vi "SDG60ConfModulation.vi"(0 "VISA resource name":refnum<visa-resource-name>="USB0::0xF4EC::0x1101::SDG6XEBC5R0119::INSTR", 1 "Modulation Type (0: AM)":u16(ring) items=["AM", "FM", "PM", "PWM", "DSBAM", "ASK", "FSK", "PSK", "CARR"], 2 "Channel (1:Channel 1)":i32(ring)=1 items=["Channel 1"=1, "Channel 2"=2], 11 "error in (no error)":errorcluster) -> (4 "VISA resource name out":refnum<visa-resource-name>, 15 "error out":errorcluster)   [LabVIEW 2018]
doc: "Selects the waveform shape, frequency, amplitude, offset, and phase for standard waveforms (including Sine, Square, Ramp, Pulse, DC and Arb).\n\nNotes: \nTo configure other parameters for pulse waveforms please run the Configure Pulse VI. \nTo configure noise waveform please run the Configure Noise VI.\nTo configure other parameters for arbitrary waveforms please run the Create Arbitrary Waveform. \nTo configure PRBS waveform please run the Configure PRBS Waveform VI."
panel:
  in  "Phase (0 deg)":dbl format="%#_12g"
  in  "Depth (%)":dbl=1000.0 format="%#_16g"
  in  "Frequency (1 Hz)":dbl=1000.0 format="%#_16g"
  in  "Mod wave shape (0:Sine)":u16(ring) items=["Sine", "Square", "Triangle", "Up Ramp", "Down Ramp", "Noise", "Arb"]
  in  "Internal/External (0: INT)":u16(ring) items=["Internal", "External"]
  # "Modulation will be turned on, as needed to be on to change\nsettings\nModulation not available when carrier is noise"
  # "AM:  Mode shape, freq, depth when set to external"
  # "Range: 0.001Hz-1 MHz\n11 digit precision"
  # "Range: 0-120%\n11 digit precision"
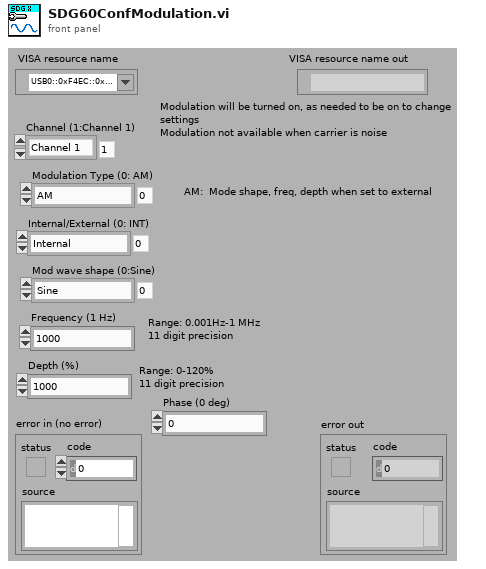
[diagram p1: front panel]
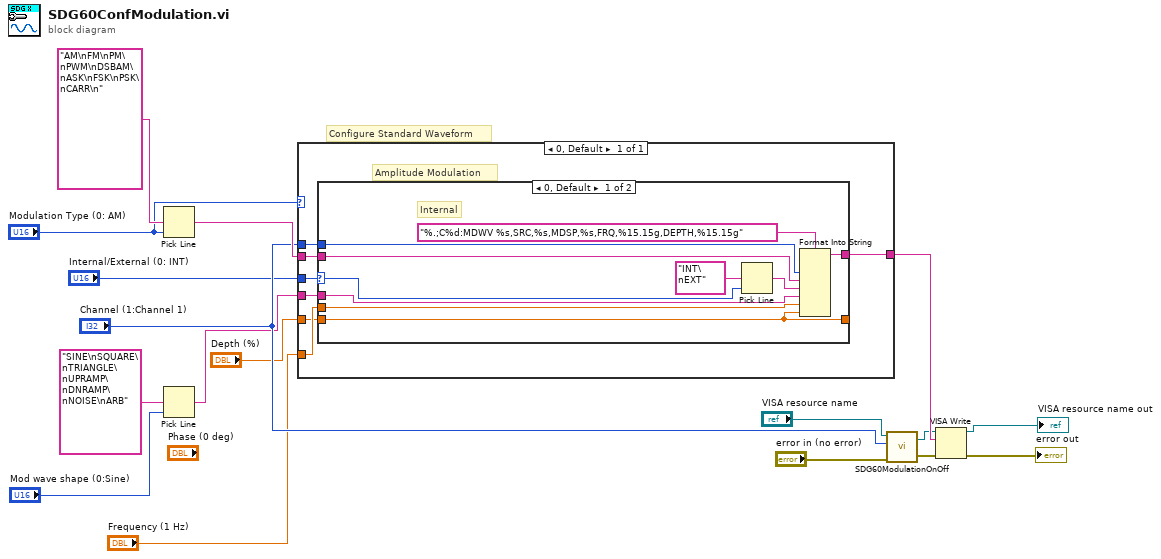
[diagram p0: block diagram]
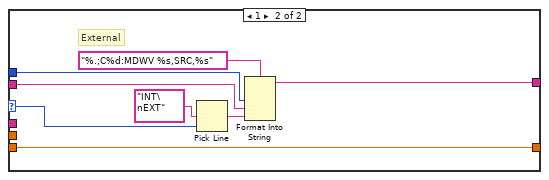
[diagram p2: hidden frame]
diagram:
  # "Configure Standard Waveform"
  n1 = Pick Line(multi-line string="AM\nFM\nPM\nPWM\nDSBAM\nASK\nFSK\nPSK\nCARR\n", line index="Modulation Type (0: AM)") -> (output string=w16:string)  [unwired: 1 in]
  n2 = Pick Line(multi-line string="SINE\nSQUARE\nTRIANGLE\nUPRAMP\nDNRAMP\nNOISE\nARB", line index="Mod wave shape (0:Sine)") -> (output string=w3:string)  [unwired: 1 in]
  n3 = case shown="0, Default" "Modulation Type (0: AM)" {
    tunnel: w16 -> [w24]
    tunnel: [w23] -> w15
    tunnel: "Channel (1:Channel 1)" -> [w22]
    tunnel: "Internal/External (0: INT)" -> [w20]
    tunnel: w3 -> [w21]
    tunnel: "Frequency (1 Hz)" -> [w19]
    tunnel: "Depth (%)" -> [w18]
    frame 0, Default {
      # "Amplitude Modulation"
      n4 = case shown="0, Default" w20 {
        selector: w20 -> [w30 w38]
        tunnel: w24 -> [w34 w42]
        tunnel: [w32 w40] -> w23
        tunnel: w22 -> [w31 w39]
        tunnel: w21 -> [w27 _]
        tunnel: w19 -> [w26 _]
        tunnel: [w25 w35] -> _
        tunnel: w18 -> [w25 w35]
        frame 0, Default {
          # "Internal"
          n5 = Pick Line(multi-line string="INT\nEXT", line index=w30) -> (output string=w29:string)  [unwired: 1 in]
          n6 = Format Into String(format string="%.;C%d:MDWV %s,SRC,%s,MDSP,%s,FRQ,%15.15g,DEPTH,%15.15g", w31, w34, w29, w27, w26, w25) -> (resulting string=w32:string)  [unwired: 2 in, 1 out]
        }
        frame 1 {
          # "External"
          n7 = Pick Line(multi-line string="INT\nEXT", line index=w38) -> (output string=w37:string)  [unwired: 1 in]
          n8 = Format Into String(format string="%.;C%d:MDWV %s,SRC,%s", w39, w42, w37) -> (resulting string=w40:string)  [unwired: 2 in, 1 out]
        }
      }
    }
  }
  n9 = call "SDG60ModulationOnOff.vi"("error in (no error)"="error in (no error)", "Channel (1: Channel1)"="Channel (1:Channel 1)", "VISA resource name"="VISA resource name") -> ("error out"=w10:errorcluster, "VISA resource name out"=w8:refnum<visa-resource-name>)  [unwired: 1 in]
  n10 = VISA Write(VISA resource name=w8, write buffer=w15, error in (no error)=w10) -> (VISA resource name out=→"VISA resource name out":refnum<visa-resource-name>, error out=→"error out":errorcluster)  [unwired: 1 out]
